vi "_Read.vi"(8 "error in (no error)":errorcluster, 11 "Fluke Multimeter in":refnum<class "Fluke Multimeter.lvclass">) -> (0 "error out":errorcluster, 2 "4 Data Points":dbl[](array[numeric]), 3 "Fluke Multimeter out":refnum<class "Fluke Multimeter.lvclass">)   [LabVIEW 2023, in "Fluke Multimeter.lvclass"]
doc: "(Protected, Dynamic) Perform a measurement and return up to four channels of data. Outsiders should not call this method, but instead the public \"Read Data.vi\"."
uses:
  Fluke Multimeter.lvclass
  Fluke Multimeter.lvclass/Fluke Multimeter.ctl
  Utility Classes/Readable/Readable.lvclass
  Fluke 8840/Fluke 8840.lvlib
panel:
  out "function (0:volts DC)":u16(ring) items=["volts DC", "volts AC", "2-wire k.ohms", "4-wire k.ohms", "mA DC", "mA AC"]
  out "range (0:auto)":u16(ring) items=["autorange", "200mV, 200 ohms", "2V, 2 kohms", "20V, 20 kohms", "200V, 200 kohms", "1000Vdc, 700 Vac, 2 Mohms", "20 Mohms"]
  out "rate (0:slow)":u16(ring) items=["slow", "medium", "fast"]
  out "trigger mode (0:internal)":u16(ring) items=["internal - continuous trigger", "external - rear panel trigger with delay", "external - bus trigger with delay", "external - rear panel trigger", "external - bus trigger"]
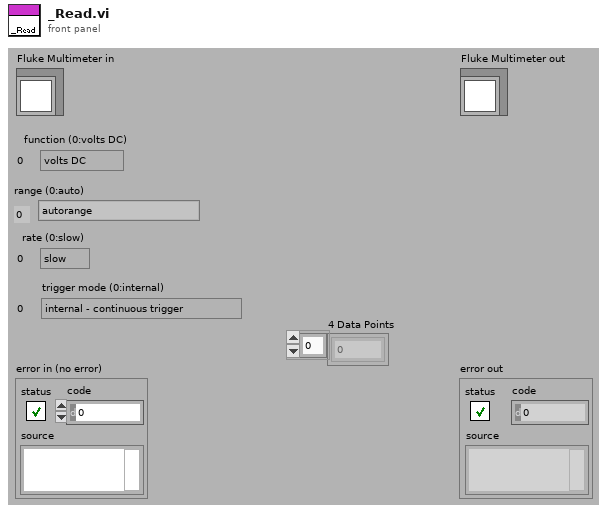
[diagram p1: front panel]
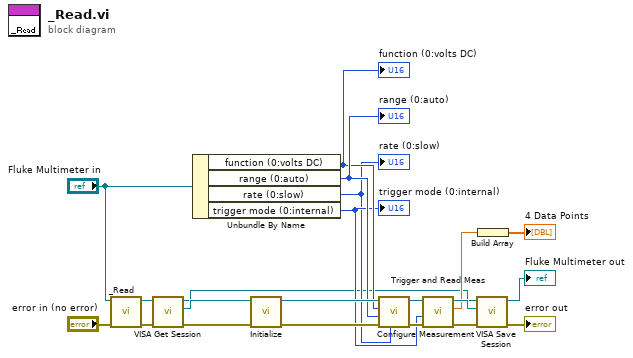
[diagram p0: block diagram]
diagram:
  n1 = call-parent "_Read.vi"("error in (no error)"="error in (no error)", "Readable in"="Fluke Multimeter in") -> ("error out"=w10:errorcluster, "Readable out"=w15:refnum<class "Fluke Multimeter.lvclass">)  [unwired: 8 out]
  n2 = call-dynamic "VISA Get Session.vi"("error in (no error)"=w10, "Instrument.lvclass in"=w15) -> ("error out"=w9:errorcluster, "VISA Resource Name"=w16:refnum<visa-resource-name>, "Instrument.lvclass out"=w3:refnum<class "Fluke Multimeter.lvclass">)  [unwired: 7 out]
  n3 = Unbundle By Name("Fluke Multimeter in") -> ("function (0:volts DC)"=w6:u16, "range (0:auto)"=w7:u16, "rate (0:slow)"=w4:u16, "trigger mode (0:internal)"=w5:u16)
  "function (0:volts DC)" <- w6
  "range (0:auto)" <- w7
  "rate (0:slow)" <- w4
  "trigger mode (0:internal)" <- w5
  n4 = call "Initialize.vi"("error in (no error)"=w9, "VISA resource name"=w16) -> ("error out"=w19:errorcluster, "VISA resource name out"=w20:refnum<visa-resource-name>)  [unwired: 1 in, 7 out]
  n5 = call "Configure Measurement.vi"("rate (0:slow)"=w4, "error in (no error)"=w19, "range (0:auto)"=w7, "function (0:volts DC)"=w6, "VISA resource name"=w20) -> ("error out"=w17:errorcluster, "VISA resource name out"=w18:refnum<visa-resource-name>)  [unwired: 5 out]
  n6 = call "Trigger and Read Meas.vi"("error in (no error)"=w17, "trigger mode (0:internal)"=w5, "VISA resource name"=w18) -> ("error out"=w13:errorcluster, "measurement"=w12:dbl, "VISA resource name out"=w14:refnum<visa-resource-name>)  [unwired: 6 out]
  n7 = call-dynamic "VISA Save Session.vi"("error in (no error)"=w13, "VISA Resource Name"=w14, "Instrument.lvclass in"=w3) -> ("error out"=→"error out":errorcluster, "Instrument.lvclass out"=→"Fluke Multimeter out":refnum<class "Fluke Multimeter.lvclass">)  [unwired: 7 out]
  n8 = Build Array(w12) -> (→"4 Data Points":dbl[])
